vi "gyro.vi"() -> (3 "x 3":dbl)   [LabVIEW 2019]
panel:
  in  "p":dbl=0.02
  in  "x":dbl=0.18
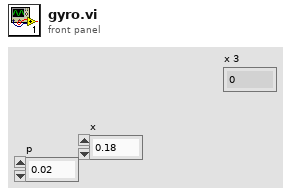
[diagram p1: front panel]
types:
  T1 = typedef "WPI_GyroDevRef.ctl" = cluster{"DevStatus":errorcluster, "Analog Channel":T2, "Gain (VoltsPerDegree/Second)":dbl, "Gyro Type":enum16{"Analog", "XRS450"}, "Handle":i32, "SPI Bus":T3, "Device Found":bool, "Sample Rate":dbl, "Calibrate On Open":bool, "Offset":dbl}
  T2 = typedef "FPGA_AIChannel.ctl" = enum8{"AI 0", "AI 1", "AI 2", "AI 3", "AI MXP 0", "AI MXP 1", "AI MXP 2", "AI MXP 3", "Invalid"}
  T3 = typedef "spi_bus.ctl" = enum16{"SPI On-Board, CS0", "SPI On-Board, CS1", "SPI On-Board, CS2", "SPI On-Board, CS3", "SPI MXP", "Invalid"}
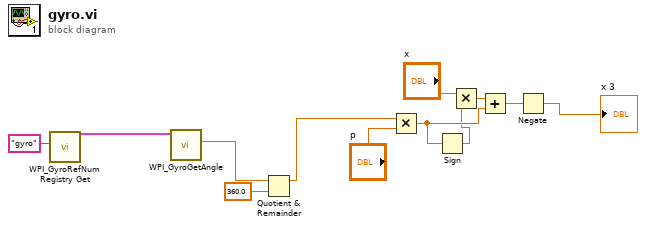
[diagram p0: block diagram]
diagram:
  n1 = call <vilib>:"WPI_GyroRefNum Registry Get.vi"("refnum name"="gyro") -> ("GyroDevRef"=w4:T1)  [unwired: 9 in, 1 out]
  n2 = call <vilib>:"WPI_GyroGetAngle.vi"("GyroDevRef"=w4) -> ("Angle"=w3:dbl)  [unwired: 6 in, 4 out]
  n3 = Quotient & Remainder(x=w3, y=360.0) -> (x-y*floor(x/y)=w1:dbl)  [unwired: 1 out]
  n4 = Multiply(x=w1, y="p") -> (x*y=w10:dbl)
  n5 = Sign(1:w10) -> (0:w6:dbl)
  n6 = Multiply(x="x", y=w6) -> (x*y=w8:dbl)
  n7 = Add(x=w8, y=w10) -> (x+y=w7:dbl)
  n8 = Negate(x=w7) -> (-x=→"x 3":dbl)
